vi "Get Tunnel Direction_Flat Sequence.vi"(7 "Tunnel Type":enum16{"Tunnel", "FlatSeqInner", "FlatSeqOuter"}(ring), 10 "FlatSeqOutTun Refnum":refnum<vi>, 11 "FlatSeqInTun Refnum":refnum<vi>) -> (3 "Tunnel Direction":enum16{"In-Going", "Out-Going"}(ring))   [LabVIEW 2023]
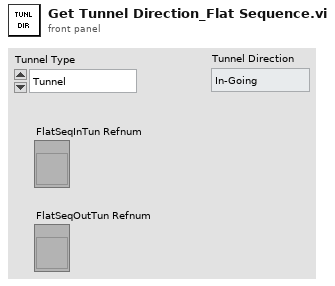
[diagram p1: front panel]
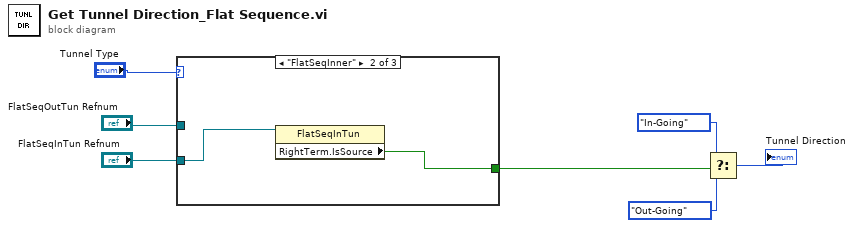
[diagram p0: block diagram]
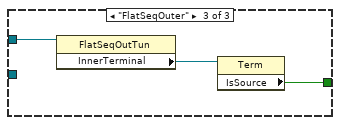
[diagram p3: hidden frame]
diagram:
  n1 = case shown="\"FlatSeqInner\"" "Tunnel Type" {
    tunnel: "FlatSeqOutTun Refnum" -> [_ _ w12]
    tunnel: "FlatSeqInTun Refnum" -> [_ w9 _]
    tunnel: [_ w8 w10] -> w1
    frame "Tunnel", Default {
    }
    frame "FlatSeqInner" {
      n2 = property class="FlatSeqInTun"(reference=w9) -> ("RightTerm.IsSource"=w8:bool)  [unwired: 1 in, 2 out]
    }
    frame "FlatSeqOuter" {
      n3 = property class="FlatSeqOutTun"(reference=w12) -> ("InnerTerminal"=w11:refnum<vi>)  [unwired: 1 in, 2 out]
      n4 = property class="Term"(reference=w11) -> ("IsSource"=w10:bool)  [unwired: 1 in, 2 out]
    }
  }
  n5 = Select(t=enum16{"In-Going", "Out-Going"}."In-Going" ("Tunnel Direction"), s=w1, f=enum16{"In-Going", "Out-Going"}."Out-Going" ("Tunnel Direction")) -> (s? t:f=→"Tunnel Direction":enum16{"In-Going", "Out-Going"})
